vi "Get Block Data Refs.vi"(8 "error in (no error)":errorcluster, 10 "Device Ref in":T1=18446744073709551615 format="%.0x", 11 "State Vars":T2 {"CompiledSettings"."Result Ch Data Refs" format="%.0x"; "CompiledSettings"."Parameter Block Data Refs"."Data Reference" format="%.0x"}) -> (0 "error out":errorcluster, 1 "Create Params Block Refs Error":errorcluster, 2 "Create Results Block Refs Error":errorcluster, 3 "State Vars out":T2 {"CompiledSettings"."Result Ch Data Refs" format="%.0x"; "CompiledSettings"."Parameter Block Data Refs"."Data Reference" format="%.0x"})   [LabVIEW 2015, in "Waveform-Processing-Custom-Device Engine.lvlib"]
uses:
  Waveform-Processing-Custom-Device Engine.lvlib
  <vilib>/NI VeriStand/Custom Device API/Custom Device API.lvlib
  <vilib>/NI Veristand/Custom Device API/Data Access Type.ctl
  Types/Async FIFOs.ctl
  <vilib>/NI Veristand/Custom Device API/Custom Device Item Ref.ctl
  Shared/CompiledSettings.ctl
  Shared/Waveform-Processing-Custom-Device Shared.lvlib
  Types/Inline State Vars.ctl
  Built/Waveform-Processing-Custom-Device/Waveform-Processing-Custom-Device Engine Windows.llb/Data Reference.ctl
  <vilib>/NI Veristand/Custom Device API/Block Data Reference.ctl
  <vilib>/NI Veristand/Custom Device API/Waveform Data Reference.ctl
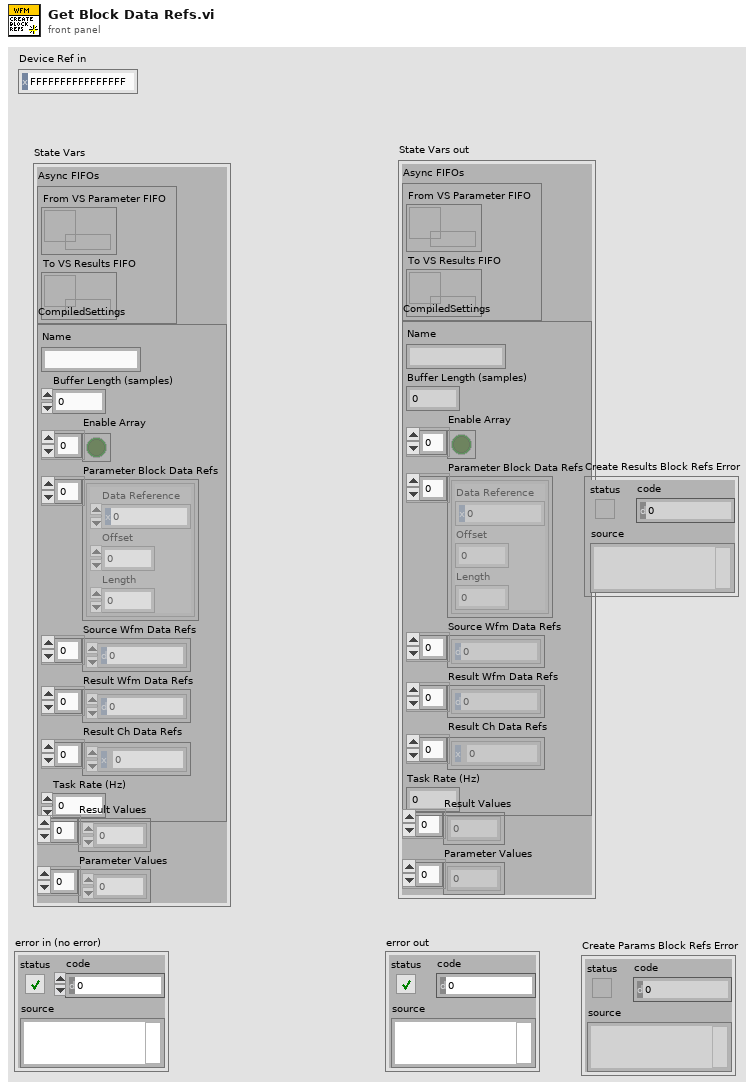
[diagram p1: front panel]
types:
  T1 = typedef "Custom Device API.lvlib/Custom Device Item Ref.ctl" = u64
  T2 = typedef "Waveform-Processing-Custom-Device Engine.lvlib/Inline State Vars.ctl" = cluster{"Async FIFOs":T3, "CompiledSettings":T4, "Result Values":dbl[], "Parameter Values":dbl[]}
  T3 = typedef "Waveform-Processing-Custom-Device Engine.lvlib/Async FIFOs.ctl" = cluster{"From VS Parameter FIFO":refnum<k33>, "To VS Results FIFO":refnum<k33>}
  T4 = typedef "Waveform-Processing-Custom-Device Shared.lvlib/CompiledSettings.ctl" = cluster{"Name":string, "Buffer Length (samples)":u32, "Enable Array":bool[], "Parameter Block Data Refs":T5[], "Source Wfm Data Refs":T7[], "Result Wfm Data Refs":T7[], "Result Ch Data Refs":T6[], "Task Rate (Hz)":dbl}
  T5 = typedef "Custom Device API.lvlib/Block Data Reference.ctl" = cluster{"Data Reference":T6, "Offset":u64, "Length":u64}
  T6 = typedef "Custom Device API.lvlib/Data Reference.ctl" = i32
  T7 = typedef "Custom Device API.lvlib/Waveform Data Reference.ctl" = i32
  T8 = typedef "Custom Device API.lvlib/Data Access Type.ctl" = enum16{"Read", "Write"}
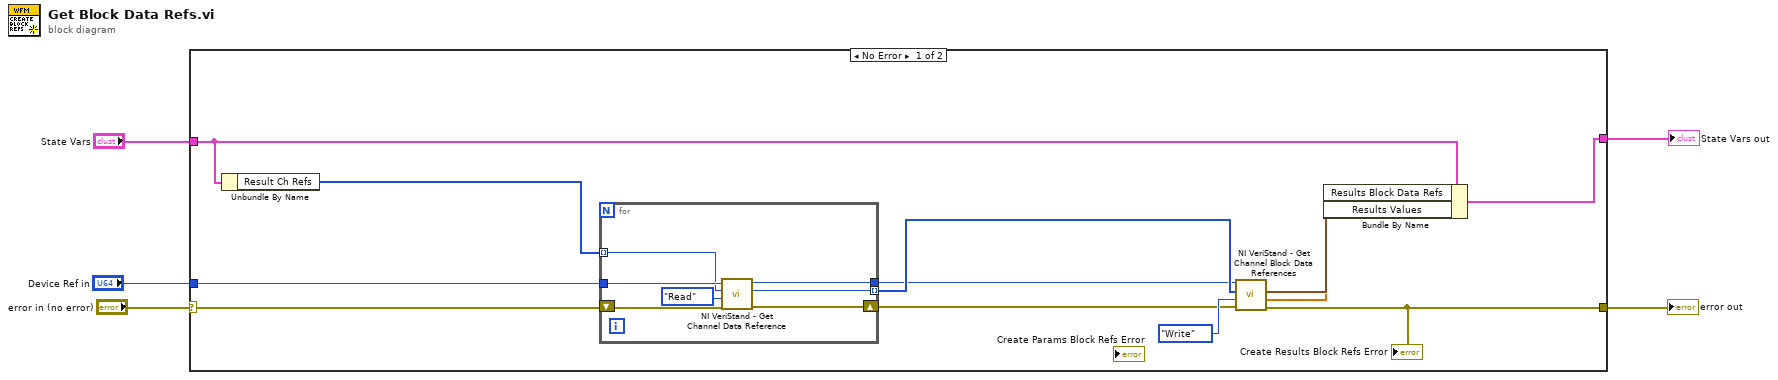
[diagram p0: block diagram]
diagram:
  n1 = case shown="No Error" "error in (no error)" {
    selector: "error in (no error)" -> [w10 w26]
    tunnel: "State Vars" -> [w17 w25]
    tunnel: [w16 w26] -> w3
    tunnel: [w14 w25] -> w2
    tunnel: "Device Ref in" -> [w11 _]
    frame No Error {
      n2 = Unbundle By Name(w17) -> ("Result Ch Refs"=w9:T1[])
      n3 = for {
        tunnel: w11 -> [w23]
        tunnel: [w20] -> w6
        tunnel: [w19] -> w8 mode=indexing
        tunnel: w9 -> [w18] mode=indexing
        shift-right: [w21] -> w7
        shift-left: w10 -> [w24]
        n4 = call <vilib>:"NI VeriStand - Get Channel Data Reference.vi"("error in (no error)"=w24, "Access"=Data_Access_Type."Read", "Channel Ref in"=w18, "Device Ref in"=w23) -> ("error out"=w21:errorcluster, "Channel Data Reference"=w19:T6, "Device Ref out"=w20:T1)  [unwired: 5 in]
      }
      n5 = call <vilib>:"NI VeriStand - Get Channel Block Data References.vi"("error in (no error)"=w7, "Access"=Data_Access_Type."Write", "Channel Refs"=w8, "Device Ref in"=w6) -> ("error out"=w16:errorcluster, "Values Array"=w12:dbl[], "Block Data Refs"=w13:T5[])  [unwired: 4 in, 1 out]
      "Create Results Block Refs Error" <- w16
      n6 = Bundle By Name(cluster=w17, "Results Block Data Refs"=w13, "Results Values"=w12) -> (w14:T2)
    }
    frame Error {
    }
  }
  "error out" <- w3
  "State Vars out" <- w2
